vi "ReadTestInfo.vi"(8 "error in":errorcluster, 11 "Path":path) -> (0 "error out":errorcluster, 2 "RunTimes":string[](array[string]), 3 "Test Information":T1={"APU Part Number:"="", "Model:"="", "Serial Number:"="", "Customer:"="", "Work Order:"="", "Pre or Post SB"="", "Run Count"=0, "APU Selected"="<Select>"} {"Run Count" min=0 step=1}, 5 "report ref":refnum<class "NI_report.lvclass">)   [LabVIEW 2018, in "File IO.lvlib"]
uses:
  File IO.lvlib
  Controller (Host)/Public Controls/Test Information.ctl
  Controller (Host)/Public VIs/PreorPostSB.ctl
  Controller (Host)/Public Controls/APU Select.ctl
  <vilib>/Utility/NIReport.llb/NI_report.lvclass
  <vilib>/Utility/NIReport.llb/Report Type.ctl
  Public Controls/Report Sheet Names.ctl
  <vilib>/addons/_office/excel.llb/Excel Get Data ([str]).vi
  Controller (Host)/Controller (Host).lvlib
  <vilib>/Utility/NIReport.llb/Excel/NI_Excel.lvclass
  <vilib>/addons/_office/NI_ReportGenerationToolkit.lvlib
  <vilib>/Utility/NIReport.llb/NI_ReportGenerationCore.lvlib
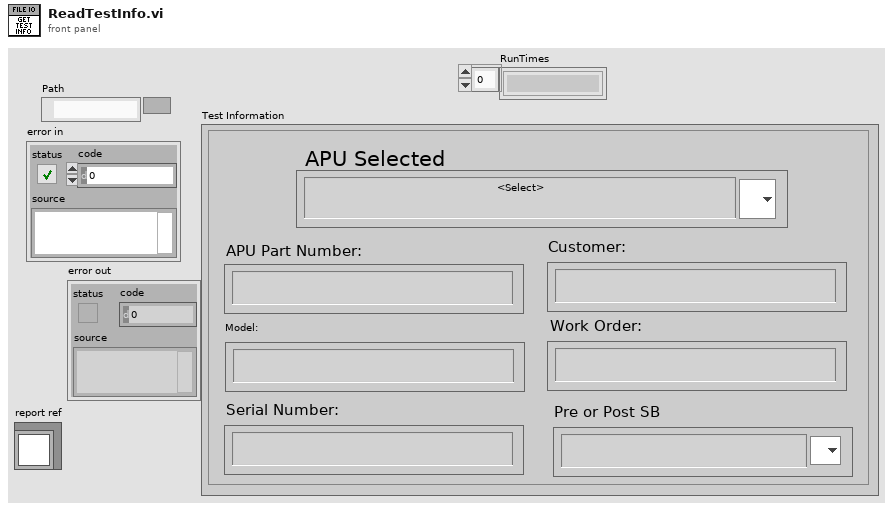
[diagram p1: front panel]
types:
  T1 = typedef "Controller (Host).lvlib/Test Information.ctl" = cluster{"APU Part Number:":string, "Model:":string, "Serial Number:":string, "Customer:":string, "Work Order:":string, "Pre or Post SB":T2, "Run Count":i32, "APU Selected":T3}
  T2 = typedef "Controller (Host).lvlib/PreorPostSB.ctl" = string
  T3 = typedef "Controller (Host).lvlib/APU Select.ctl" = string
  T4 = typedef "File IO.lvlib/Report Sheet Names.ctl" = string
  T5 = typedef "NI_ReportGenerationCore.lvlib/Report Type.ctl" = enum16{"HTML", "Word", "Excel"}
  T6 = enum16{"maximized", "minimized", "normal", "no change"}
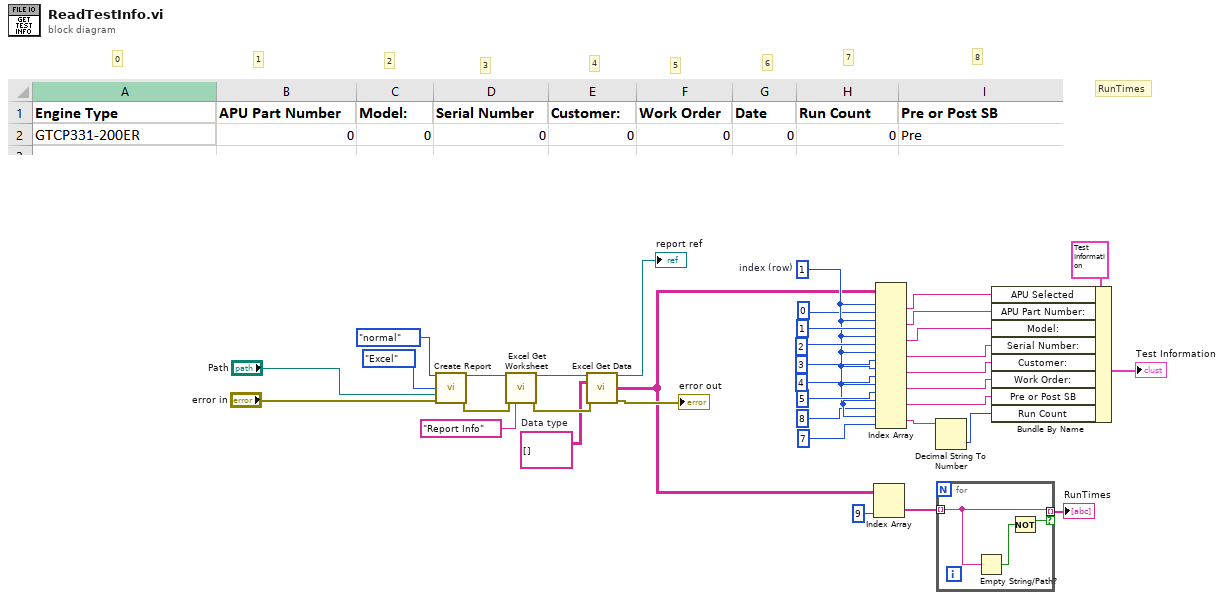
[diagram p0: block diagram]
diagram:
  w13 = 1  # index (row)
  w29 = string[][] []  # Data type
  # "RunTimes"
  # "0"
  # "8"
  # "7"
  # "6"
  # "5"
  # "4"
  # "3"
  # "2"
  # "1"
  n1 = call <vilib>:"Create Report.vi"("window state (normal)"=T6."normal", "report type"=Report_Type."Excel", "template (empty)"="Path", "error in (no error)"="error in") -> ("report out"=w32:refnum<class "NI_report.lvclass">, "error out"=w31:errorcluster)  [unwired: 10 in]
  n2 = call <vilib>:"Excel Get Worksheet.vi"("report in"=w32, "error in (no error)"=w31, "name (\"\")"=T4 "Report Info" ("Sheet Name")) -> ("report out"=w34:refnum<class "NI_report.lvclass">, "error out"=w35:errorcluster)  [unwired: 11 in]
  n3 = call-poly <vilib>:"Excel Get Data.vi"("report in"=w34, "data type"=w29, "error in (no error)"=w35) -> ("report out"=→"report ref":refnum<class "NI_report.lvclass">, "data"=w4:string[][], "error out"=→"error out":errorcluster)  [unwired: 10 in]
  n4 = Index Array(array=w4, index (col)=9 ("disabled index (col)")) -> (element=w2:string[])  [unwired: 1 in]
  n5 = Index Array(array=w4, index (row) #1=w13, index (col) #1=0 ("disabled index (col)"), index (row) #2=w13, index (col) #2=1 ("disabled index (col)"), index (row) #3=w13, index (col) #3=2 ("disabled index (col)"), index (row) #4=w13, index (col) #4=3 ("disabled index (col)"), index (row) #5=w13, index (col) #5=4 ("disabled index (col)"), index (row) #6=w13, index (col) #6=5 ("disabled index (col)"), index (row) #7=w13, index (col) #7=8 ("disabled index (col)"), index (row) #8=w13, index (col) #8=7 ("disabled index (col)")) -> (element #1=w11:string, element #2=w23:string, element #3=w18:string, element #4=w17:string, element #5=w16:string, element #6=w15:string, element #7=w6:string, element #8=w5:string)
  n6 = Decimal String To Number(string=w5) -> (number=w14:i32)  [unwired: 2 in, 1 out]
  n7 = for {
    tunnel: w2 -> [w39] mode=indexing
    tunnel: [w39] -> w1 mode=indexing if=w37
    n8 = Empty String/Path?(string/path=w39) -> (empty?=w38:bool)
    n9 = Not(x=w38) -> (.not. x?=w37:bool)
  }
  "RunTimes" <- w1
  n10 = Bundle By Name(cluster=T1 {"APU Part Number:"="", "Model:"="", "Serial Number:"="", "Customer:"="", "Work Order:"="", "Pre or Post SB"="", "Run Count"=0, "APU Selected"="<Select>"} ("Test Information"), "APU Selected"=w11, "APU Part Number:"=w23, "Model:"=w18, "Serial Number:"=w17, "Customer:"=w16, "Work Order:"=w15, "Pre or Post SB"=w6, "Run Count"=w14) -> (→"Test Information":T1)
